vi "Rotate Degrees.vi"(11 "Degrees":dbl=30.0 format="%#_13g") -> ()   [LabVIEW 2015]
doc: "Assumes that + rotation is clockwise and - is counterclockwise"
uses:
  Sprocket/src/Action/Action Name.ctl
  Sprocket/src/Refname/Refname to String (Actuator).vi
  Sprocket/src/Refname/Actuators.ctl
  Sprocket/lib/Sprocket.lvlib
panel:
  in  "Rotate Speed":dbl=0.6
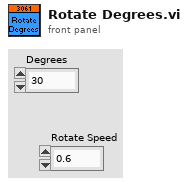
[diagram p1: front panel]
types:
  T1 = typedef "Sprocket.lvlib/Action Name.ctl" = enum16{"No Action", "Drive Train Left", "Drive Train Right", "Drive Train Both", "Collector Motor Roll", "Collector Motor Eject", "Collector Motor Collect", "Collector Motor Stop", "Collector Extend", "Collector Retract", "Shifter High", "Shifter Low", "Collector Motor Stall", "Wedge Roll"}
  T2 = typedef "Sprocket.lvlib/Actuators.ctl" = enum16{"Drive Motor 1 (R)", "Drive Motor 2 (R)", "Drive Motor 3 (R)", "Drive Motor 4 (L)", "Drive Motor 5 (L)", "Drive Motor 6 (L)", "Collector Motor", "Collector Solenoid", "Compressor", "SonicShifter", "Gyro", "UltraSonic Front Left", "UltraSonic Back Left", "Wedge Motor", "Wedge LS"}
  T3 = typedef "WPI_GyroDevRef.ctl" = cluster{"DevStatus":errorcluster, "Analog Channel":T4, "Offset":dbl, "Gain (VoltsPerDegree/Second)":dbl, "Gyro Type":enum16{"Analog", "XRS450"}, "Handle":i32, "SPI Bus":T5, "Device Found":bool, "Sample Rate":dbl, "Calibrate On Open":bool}
  T4 = typedef "FPGA_AIChannel.ctl" = enum8{"AI 0", "AI 1", "AI 2", "AI 3", "AI MXP 0", "AI MXP 1", "AI MXP 2", "AI MXP 3", "Invalid"}
  T5 = typedef "spi_bus.ctl" = enum16{"SPI On-Board, CS0", "SPI On-Board, CS1", "SPI On-Board, CS2", "SPI On-Board, CS3", "SPI MXP", "Invalid"}
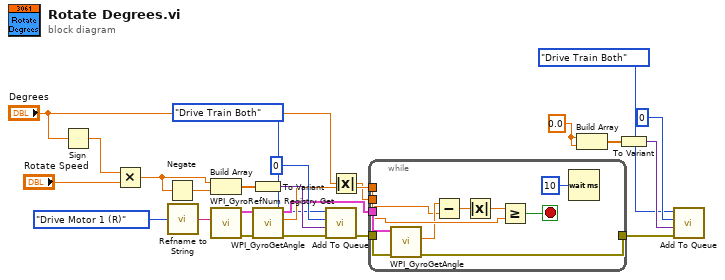
[diagram p0: block diagram]
diagram:
  w19 = 0.0
  n1 = Sign(1:"Degrees") -> (0:w15:dbl)
  n2 = Multiply(x=w15, y="Rotate Speed") -> (x*y=w14:dbl)
  n3 = Negate(x=w14) -> (-x=w13:dbl)
  n4 = call-poly "Refname to String.vi"("Actuator Refname"=Actuators."Drive Motor 1 (R)") -> ("Refnum Name"=w24:string)
  n5 = Build Array(w14, w13) -> (w16:dbl[])
  n6 = call <vilib>:"WPI_GyroRefNum Registry Get.vi"("refnum name"=w24) -> ("error out"=w6:errorcluster, "GyroDevRef"=w23:T3)  [unwired: 9 in]
  n7 = To Variant(anything=w16) -> (Variant=w17:variant)
  n8 = call <vilib>:"WPI_GyroGetAngle.vi"("error in (no error)"=w6, "GyroDevRef"=w23) -> ("error out"=w5:errorcluster, "Angle"=w7:dbl, "GyroDevRef"=w8:T3)  [unwired: 6 in, 1 out]
  n9 = call "Add To Queue.vi"("error in"=w5, "Data"=w17, "Priority"=0, "Action"=Action_Name."Drive Train Both") -> ("error out"=w10:errorcluster)  [unwired: 7 in]
  n10 = Absolute Value(x="Degrees") -> (abs(x)=w4:dbl)
  n11 = while {
    tunnel: w8 -> [w34]
    tunnel: w4 -> [w31]
    tunnel: w10 -> [w27]
    tunnel: [w26] -> w9
    tunnel: w7 -> [w29]
    stop <- w32 stop-if-true
    n12 = call <vilib>:"WPI_GyroGetAngle.vi"("error in (no error)"=w27, "GyroDevRef"=w34) -> ("error out"=w26:errorcluster, "Angle"=w30:dbl)  [unwired: 6 in, 2 out]
    n13 = Subtract(x=w30, y=w29) -> (x-y=w28:dbl)
    n14 = Absolute Value(x=w28) -> (abs(x)=w33:dbl)
    n15 = Greater Or Equal?(x=w33, y=w31) -> (x >= y?=w32:bool)
    n16 = Wait (ms)(milliseconds to wait=u32 10) -> ()  [unwired: 1 out]
  }
  n17 = Build Array(w19, w19) -> (w22:dbl[])
  n18 = To Variant(anything=w22) -> (Variant=w21:variant)
  n19 = call "Add To Queue.vi"("error in"=w9, "Data"=w21, "Priority"=0, "Action"=Action_Name."Drive Train Both") -> ()  [unwired: 7 in, 1 out]
